vi "PSP-Nx-Direct.vi"() -> ()   [LabVIEW 2009]
uses:
  <vilib>/NXT/Block Support/NXT_InputPort.ctl
panel:
  out "Right Y:":u8=127
  out "Right  X:":u8=128
  out "Left Y":u8=128
  out "Left  X":u8=128
  out "R 3":bool
  out "L 3":bool
  out "R 2":bool
  out "L 1":bool
  out "R 1":bool
  out "L 2":bool
  out "Start":bool
  out "Select":bool
  out "R":bool
  out "U":bool
  out "L":bool
  out "D":bool
  out "[]":bool
  out "O":bool
  out "^":bool
  out "X":bool
  in  "stop":bool
  in  "Select your \nInput Port":T1 items=["Port 1", "Port 2", "Port 3", "Port 4"]
  in  "Select your \nDevice Address":u8=2
  # "mindsensors.com\nCopyright (c) 2009 by mindsensors.com\nEmail: info (<at>) mindsensors (<dot>) com\n\nThis program is free software. You can redistribute it and/or modify\nit under the terms of the GNU General Public License as published by\nthe Free Software Foundation; version 3 of the License.\nRead the license at: http://www.gnu.org/licenses/gpl.txt"
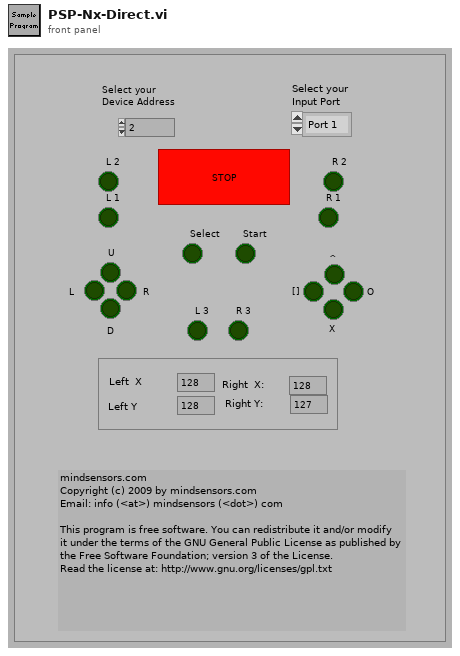
[diagram p1: front panel]
types:
  T1 = typedef "NXT_InputPort.ctl" = u8
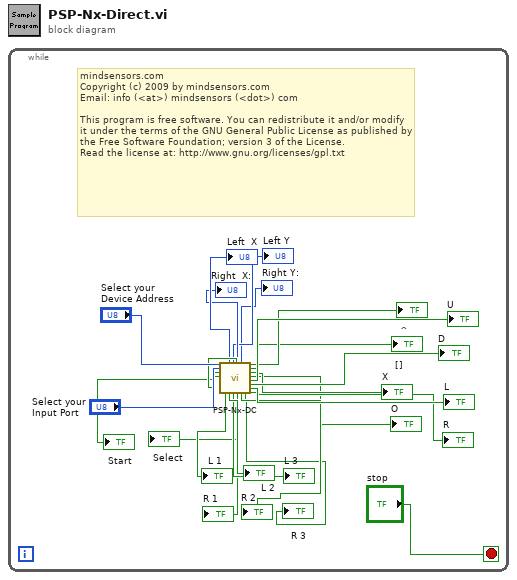
[diagram p0: block diagram]
diagram:
  n1 = while {
    stop <- "stop" stop-if-true
    # "mindsensors.com\nCopyright (c) 2009 by mindsensors.com\nEmail: info (<at>) mindsensors (<dot>) com\n\nThis program is free software. You can redistribute it and/or modify\nit under the terms of the GNU General Public License as published by\nthe Free Software Foundation; version 3 of the License.\nRead the license at: http://www.gnu.org/licenses/gpl.txt"
    n2 = call "PSP-Nx-DC.vi"("Select your \nDevice Address"="Select your \nDevice Address", "Select your \nInput Port"="Select your \nInput Port") -> ("Select"=→"Select":bool, "Start"=→"Start":bool, "L 1"=→"L 1":bool, "Left  X"=→"Left  X":u8, "L 2"=→"L 2":bool, "Left Y"=→"Left Y":u8, "L 3"=→"L 3":bool, "Right  X:"=→"Right  X:":u8, "R 1"=→"R 1":bool, "Right Y:"=→"Right Y:":u8, "R 2"=→"R 2":bool, "R 3"=→"R 3":bool, "^"=→"^":bool, "[]"=→"[]":bool, "X"=→"X":bool, "O"=→"O":bool, "UP"=→"U":bool, "DOWN"=→"D":bool, "LEFT"=→"L":bool, "RIGHT"=→"R":bool)  [unwired: 5 in, 1 out]
  }
